vi "Orphaned Pointer Test.vi"() -> ()   [LabVIEW 2020, in "Test Executive.lvlib"]
uses:
  <vilib>/gpm_packages/@cs/test-executive/Source/Test Executive/Test Executive.lvlib
  <vilib>/gpm_packages/@cs/test-executive/Source/Test Executive/TestExecutive/Test Executive.lvclass
  C:/Program Files/National Instruments/LabVIEW 2020/vi.lib/gpm_packages/@cs/test-executive/Source/Test Executive/ITestExecutive/ITest Executive.lvclass
  535d4302-c68f-4885-a44b-9fd21cc49a13.vi
  d56c1b87-d15c-4ae1-ada6-9dea4e4e1ece.vi
  59772425-59e7-4f66-baa3-1318a0611b1e.vi
  760e66ce-c946-441b-ad01-bb06bd553242.vi
  <vilib>/Utility/error.llb/Error Cluster From Error Code.vi
  <vilib>/gpm_packages/@cs/test-executive/Source/Test Executive/ITestExecutive/ITest Executive.lvclass
  <vilib>/gpm_packages/@cs/test-executive/Source/Test Executive/TestExecutive Ref/TestExecutive Ref.lvclass
panel:
  in  "Tree Post Remove":string(tree)
  out "Orphaned Pointer IDs":string[](array[string])
  in  "Tree":string(tree)
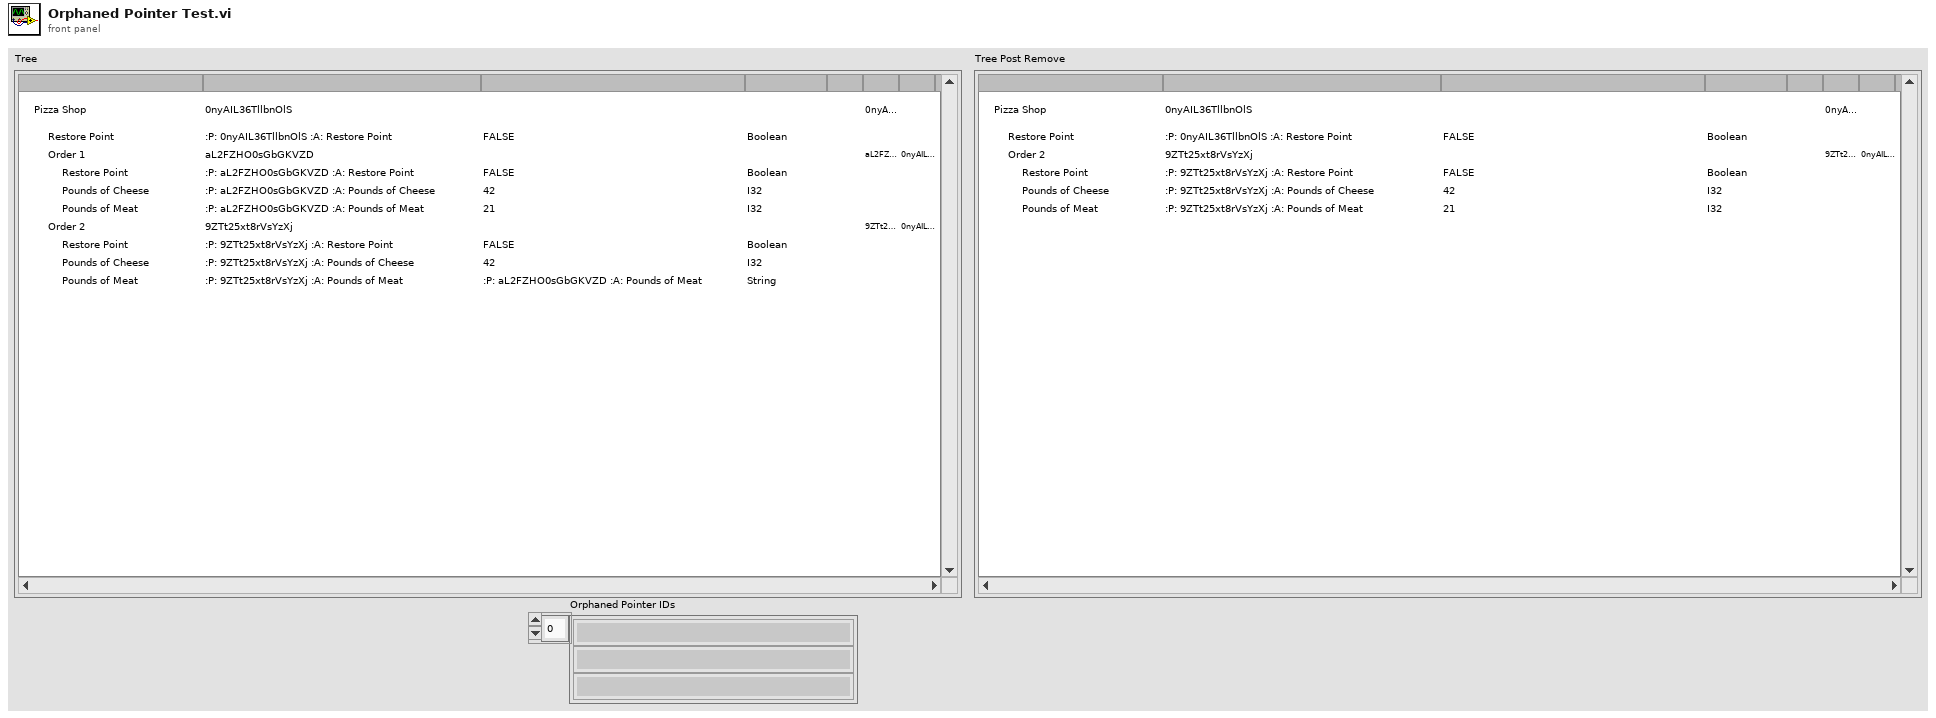
[diagram p1: front panel]
types:
  T1 = cluster{"Left Cell String":string, "Child Text":string[], "Child Tag":string, "Item Indent":i32, "Child Only?":bool, "Glyph Index":i32}[]
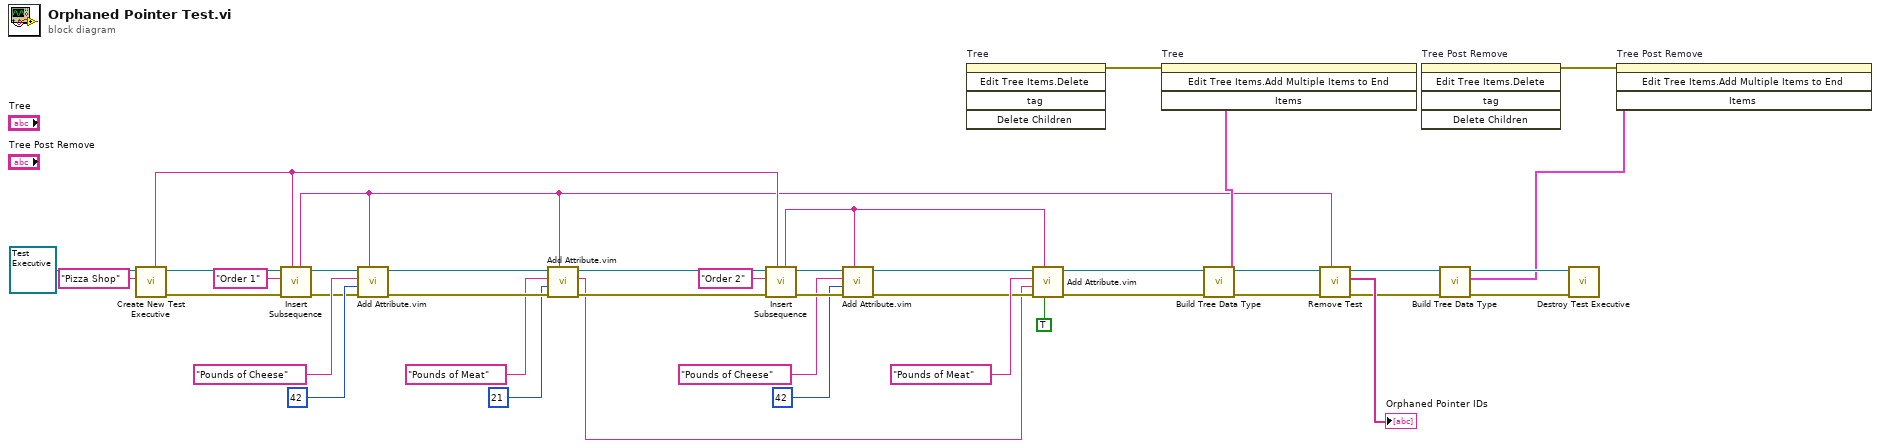
[diagram p0: block diagram]
diagram:
  n1 = call <vilib>:"Create New Test Executive.vi"("Name"="Pizza Shop", "Test Executive"=refnum<class "Test Executive.lvclass"> refnum ("Test Executive.lvlib:Test Executive.lvclass")) -> ("error out"=w38:errorcluster, "Test Executive Ref"=w39:refnum<data-value>, "Test Executive ID out"=w17:string)  [unwired: 7 in]
  n2 = call <vilib>:"Insert Subsequence.vi"("Parent ID"=w17, "error in (no error)"=w38, "Name"="Order 1", "Test Executive Ref"=w39) -> ("error out"=w33:errorcluster, "Test Executive Ref out"=w34:refnum<data-value>, "Unique ID out"=w8:string)  [unwired: 4 in, 1 out]
  n3 = call "Add Attribute.vim"("ID"=w8, "error in (no error)"=w33, "Attribute"=42, "Attribute Name"="Pounds of Cheese", "Test Executive Ref"=w34) -> ("error out"=w31:errorcluster, "Test Executive Ref out"=w32:refnum<data-value>)  [unwired: 3 in, 2 out]
  n4 = call "Add Attribute.vim"("ID"=w8, "error in (no error)"=w31, "Attribute"=21, "Attribute Name"="Pounds of Meat", "Test Executive Ref"=w32) -> ("error out"=w18:errorcluster, "Attribute ID out"=w15:string, "Test Executive Ref out"=w19:refnum<data-value>)  [unwired: 3 in, 1 out]
  n5 = call <vilib>:"Insert Subsequence.vi"("Parent ID"=w17, "error in (no error)"=w18, "Name"="Order 2", "Test Executive Ref"=w19) -> ("error out"=w24:errorcluster, "Test Executive Ref out"=w23:refnum<data-value>, "Unique ID out"=w27:string)  [unwired: 4 in, 1 out]
  n6 = call "Add Attribute.vim"("ID"=w27, "error in (no error)"=w24, "Attribute"=42, "Attribute Name"="Pounds of Cheese", "Test Executive Ref"=w23) -> ("error out"=w26:errorcluster, "Test Executive Ref out"=w25:refnum<data-value>)  [unwired: 3 in, 2 out]
  n7 = invoke on="Tree" class="Tree (strict)" method="Edit Tree Items.Delete"() -> (error out=w12:errorcluster)  [unwired: 5 in, 4 out]
  n8 = call "Add Attribute.vim"("Pointer?"=TRUE, "ID"=w27, "error in (no error)"=w26, "Attribute"=w15, "Attribute Name"="Pounds of Meat", "Test Executive Ref"=w25) -> ("error out"=w13:errorcluster, "Test Executive Ref out"=w14:refnum<data-value>)  [unwired: 2 in, 2 out]
  n9 = call <vilib>:"Build Tree Data Type.vi"("error in (no error)"=w13, "Test Executive Ref"=w14) -> ("error out"=w9:errorcluster, "Tree Data"=w11:T1, "Test Executive Ref out"=w10:refnum<data-value>)  [unwired: 7 in]
  n10 = invoke on="Tree" class="Tree (strict)" method="Edit Tree Items.Add Multiple Items to End"(error in=w12, "Items"=w11) -> ()  [unwired: 2 in, 4 out]
  n11 = call <vilib>:"Remove Test.vi"("Test ID"=w8, "error in (no error)"=w9, "Test Executive Ref"=w10) -> ("error out"=w6:errorcluster, "Orphaned Pointer IDs"=→"Orphaned Pointer IDs":string[], "Test Executive Ref out"=w4:refnum<data-value>)  [unwired: 6 in]
  n12 = invoke on="Tree Post Remove" class="Tree (strict)" method="Edit Tree Items.Delete"() -> (error out=w2:errorcluster)  [unwired: 5 in, 4 out]
  n13 = call <vilib>:"Build Tree Data Type.vi"("error in (no error)"=w6, "Test Executive Ref"=w4) -> ("error out"=w5:errorcluster, "Tree Data"=w1:T1, "Test Executive Ref out"=w3:refnum<data-value>)  [unwired: 7 in]
  n14 = call <vilib>:"Destroy Test Executive.vi"("error in (no error)"=w5, "Test Executive Ref"=w3) -> ()  [unwired: 9 in, 1 out]
  n15 = invoke on="Tree Post Remove" class="Tree (strict)" method="Edit Tree Items.Add Multiple Items to End"(error in=w2, "Items"=w1) -> ()  [unwired: 2 in, 4 out]
